vi "Pre Launch Init.vi"(11 "InterferometryUI in":refnum<class "InterferometryUI.lvclass">) -> (0 "error out":errorcluster, 3 "InterferometryUI out":refnum<class "InterferometryUI.lvclass">)   [LabVIEW 2023, in "InterferometryUI.lvlib" / "InterferometryUI.lvclass"]
doc: "(<B>Filename</B>: Actor Framework.lvlib:Actor.lvclass:Pre Launch Init.vi)\n\nDefines behavior that occurs after the Launch Nested Actor method is invoked but before the actor's Actor Core method begins running.\n\nBy default, this method does nothing. A descendant class may override it to define behavior."
uses:
  InterferometryUI.lvclass
  <vilib>/ActorFramework/Actor/Actor.lvclass
  typedefs/instrumentType.ctl
  typedefs/typedefs.lvlib
  <vilib>/ActorFramework/Message Enqueuer/Message Enqueuer.lvclass
  ConcreteClasses/ConcreteInstrumentClasses/CameraClasses/Hama_LV/HamaCam/HamaCam/FoundInstruments.ctl
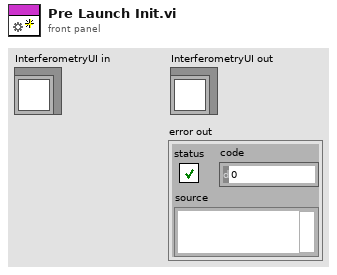
[diagram p1: front panel]
types:
  T1 = typedef "typedefs.lvlib/FoundInstruments.ctl" = cluster{"Instr Error":errorcluster, "Address":cluster{"address type":enum16{"VISA", "Index"}, "Address":string, "instrument type":T2}, "CurrentState":cluster{"Initialized":bool, "Connected":bool, "Running":bool, "Error":bool}, "Enqueuer":refnum<class "Message Enqueuer.lvclass">}[]
  T2 = typedef "typedefs.lvlib/instrumentType.ctl" = enum16{"Spectrometer", "Camera", "Stepper"}
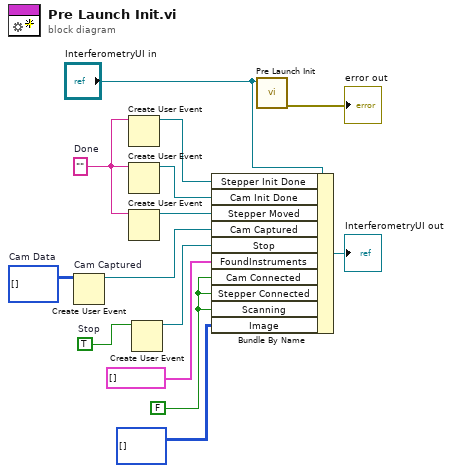
[diagram p0: block diagram]
diagram:
  w2 = u16[][] []  # Cam Data
  w4 = FALSE ("Cam Connected")
  w8 = ""  # Done
  w9 = TRUE  # Stop
  n1 = Create User Event "Cam Captured"(user event datatype=w2) -> (user event=w1:refnum<user-event>)  [unwired: 1 in, 1 out]
  n2 = Create User Event(user event datatype=w8) -> (user event=w13:refnum<user-event>)  [unwired: 1 in, 1 out]
  n3 = Create User Event(user event datatype=w8) -> (user event=w12:refnum<user-event>)  [unwired: 1 in, 1 out]
  n4 = Create User Event(user event datatype=w8) -> (user event=w11:refnum<user-event>)  [unwired: 1 in, 1 out]
  n5 = Create User Event(user event datatype=w9) -> (user event=w10:refnum<user-event>)  [unwired: 1 in, 1 out]
  n6 = Bundle By Name(cluster="InterferometryUI in", "Stepper Init Done"=w13, "Cam Init Done"=w12, "Stepper Moved"=w11, "Cam Captured"=w1, "Stop"=w10, "FoundInstruments"=T1 [], "Cam Connected"=w4, "Stepper Connected"=w4, "Scanning"=w4, "Image"=u16[][] []) -> (→"InterferometryUI out":refnum<class "InterferometryUI.lvclass">)
  n7 = call-parent "Pre Launch Init.vi"("Actor in"="InterferometryUI in") -> ("error out"=→"error out":errorcluster)  [unwired: 9 in, 1 out]
